vi "WILT Cutout Delay.vi"(6 "Delay After Cutout (sec)":dbl=5.0 format="%#_13g", 7 "Cut-In?":bool, 8 "Error In":errorcluster, 9 "Current Threshold":dbl=1.0 format="%#_13g", 10 "L2 Current":dbl, 11 "L1 Current":dbl) -> (0 "Error Out":errorcluster, 1 "Normal Trigger":bool, 2 "Elapsed Time (sec)":dbl format="%.2f", 3 "Delayed Trigger":bool)   [LabVIEW 2016]
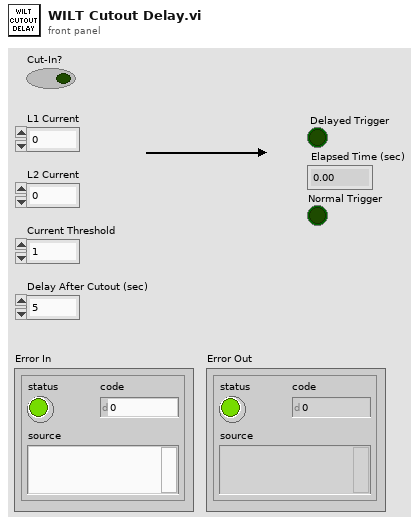
[diagram p1: front panel]
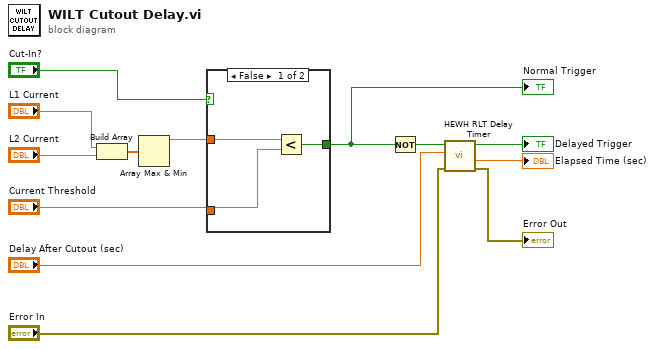
[diagram p0: block diagram]
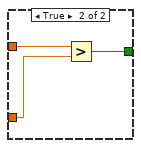
[diagram p2: hidden frame]
diagram:
  n1 = Build Array("L1 Current", "L2 Current") -> (w11:dbl[])
  n2 = Array Max & Min(array=w11) -> (max value=w9:dbl)  [unwired: 3 out]
  n3 = case shown="False" "Cut-In?" {
    tunnel: "Current Threshold" -> [w16 w18]
    tunnel: w9 -> [w15 w19]
    tunnel: [w14 w17] -> w6
    frame False {
      n4 = Less?(x=w15, y=w16) -> (x < y?=w14:bool)
    }
    frame True {
      n5 = Greater?(x=w19, y=w18) -> (0:w17:bool)
    }
  }
  "Normal Trigger" <- w6
  n6 = Not(x=w6) -> (.not. x?=w5:bool)
  n7 = call "HEWH RLT Delay Timer.vi"("Error In"="Error In", "Delay After Cutout (sec)"="Delay After Cutout (sec)", "Heat Source ON (1=ON)"=w5) -> ("Error Out"=→"Error Out":errorcluster, "Elapsed Time (sec)"=→"Elapsed Time (sec)":dbl, "Delay is Over"=→"Delayed Trigger":bool)  [unwired: 6 in]
